vi "GV count 0.vi"() -> ()   [LabVIEW 2017]
panel:
  in  "Count 0":u8
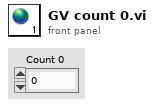
[diagram p1: front panel]
diagram:
